vi "hickey_FinalProject.vi"() -> ()   [LabVIEW 2014]
uses:
  <vilib>/MakerHub/LINX/Private/Type Defs/User Platform.ctl
  <vilib>/MakerHub/LINX/Private/Type Defs/Interface.ctl
  <vilib>/MakerHub/LINX/Public/Peripherals/Analog/Analog Read 1 Chan.vi
  <vilib>/MakerHub/LINX/Public/Peripherals/Digital/Digital Write 1 Chan.vi
  <vilib>/MakerHub/LINX/LMH-LINX.lvlib
panel:
  out "AI Value":dbl
  in  "Serial Port":refnum<visa-resource-name>="N/A"
  in  "Interface":T1
  in  "Platform":T2
  in  "stop":bool
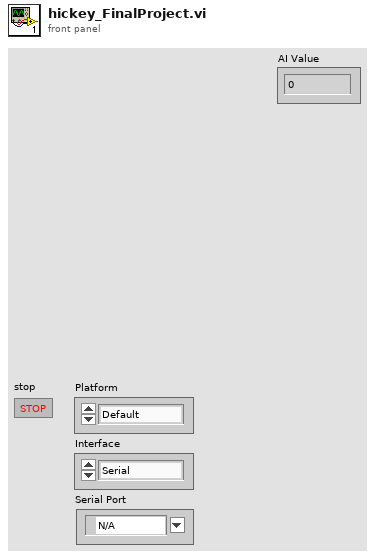
[diagram p1: front panel]
types:
  T1 = typedef "LMH-LINX.lvlib/Interface.ctl" = enum16{"Serial", "TCP"}
  T2 = typedef "LMH-LINX.lvlib/User Platform.ctl" = enum16{"Default", "LINX", "myRIO"}
  T3 = typedef "LMH-LINX.lvlib/LINX Ref.ctl" = cluster{"Platform":T4, "Interface":T1, "LINX Device Config":T5}
  T4 = typedef "LMH-LINX.lvlib/Platform.ctl" = enum16{"LINX", "myRIO"}
  T5 = typedef "LMH-LINX.lvlib/Device.lvlib/LINX Device Config.ctl" = cluster{"Interface":T1, "COM Port":refnum<visa-resource-name>, "TCP Configuration":T6, "Device Family":u8, "Device ID":u8, "Device Name":string, "TCP Ref":refnum<k5>, "Channels":T7}
  T6 = typedef "LMH-LINX.lvlib/Device.lvlib/TCP Config.ctl" = cluster{"IP Address":string, "Port":u16}
  T7 = typedef "LMH-LINX.lvlib/Channels.ctl" = cluster{"DI":u8[], "DO":u8[], "AI":u8[], "AO":u8[], "PWM":u8[], "QE":u8[], "UART":u8[], "I2C 2":u8[], "SPI":u8[], "CAN":u8[], "Servo":u8[], "AI Ref (V)":dbl, "AO Ref (V)":dbl, "AO Resolution (Bits)":u8}
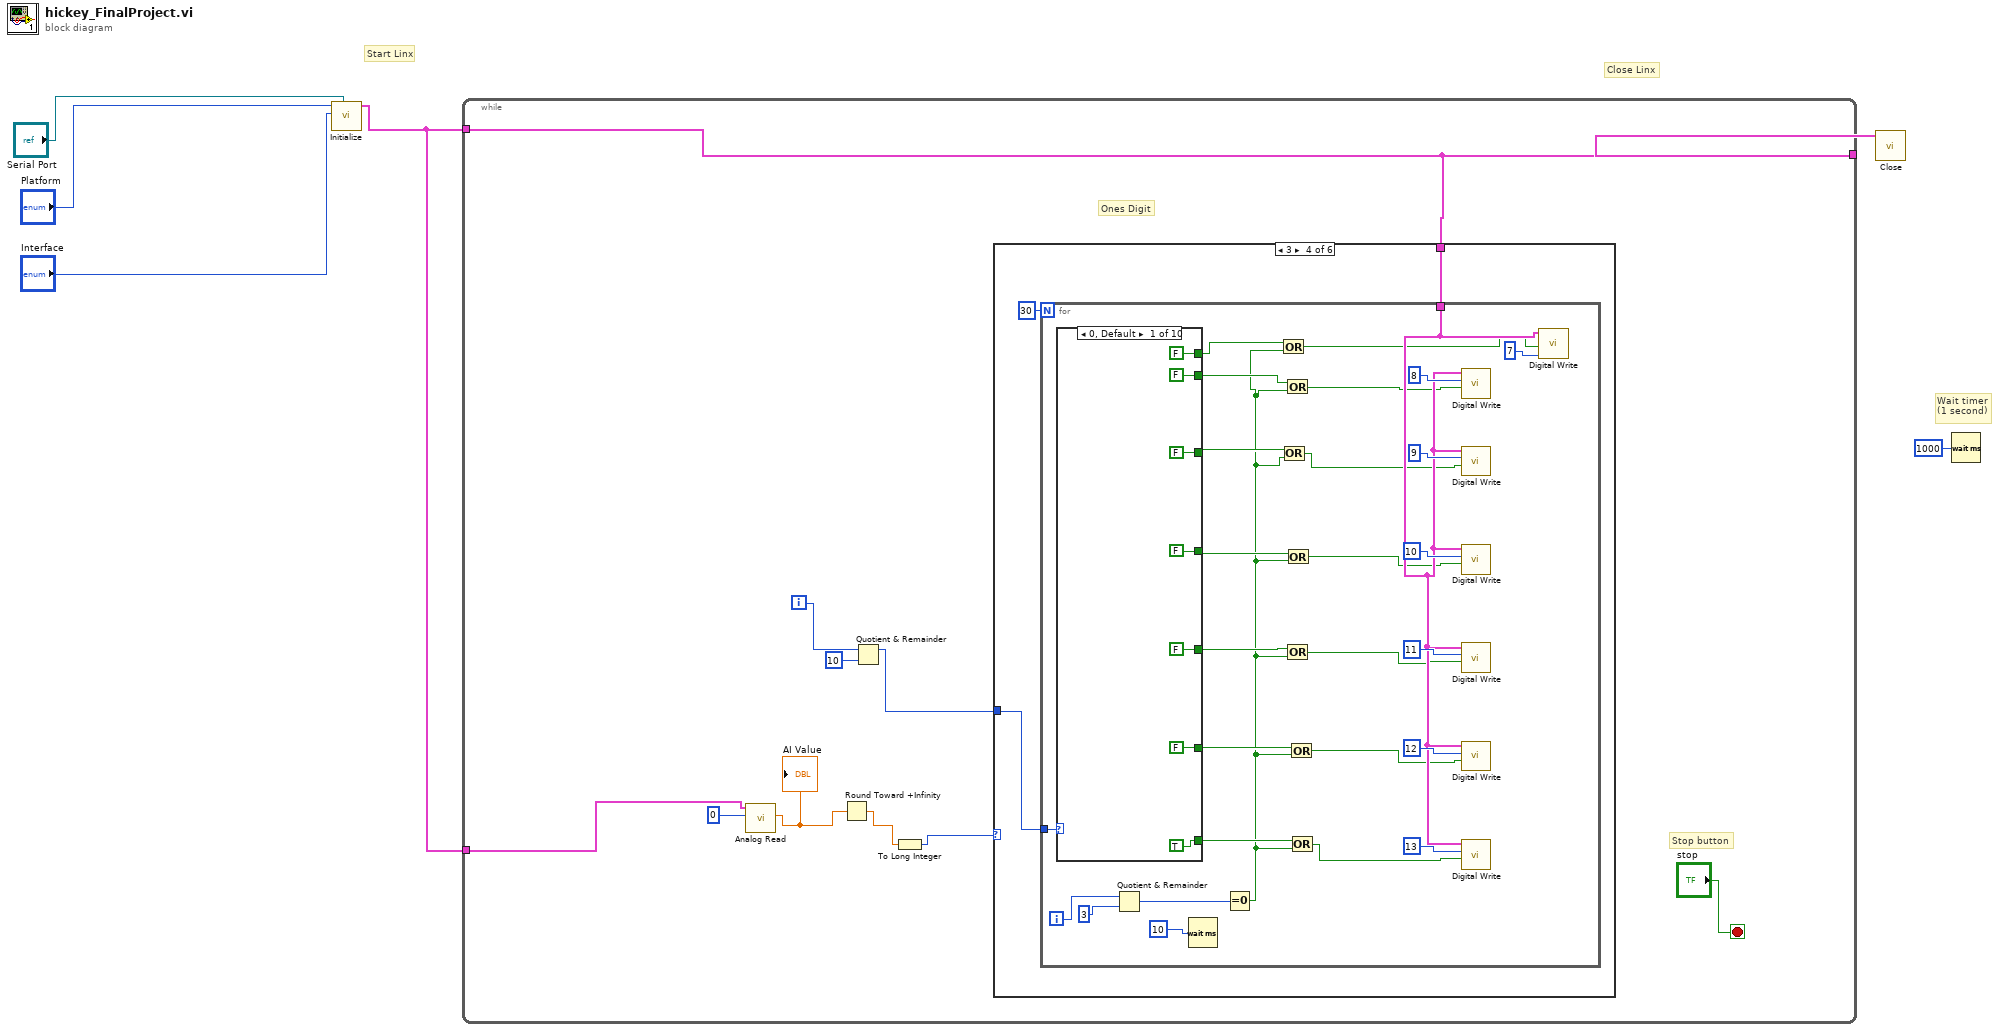
[diagram p0: block diagram]
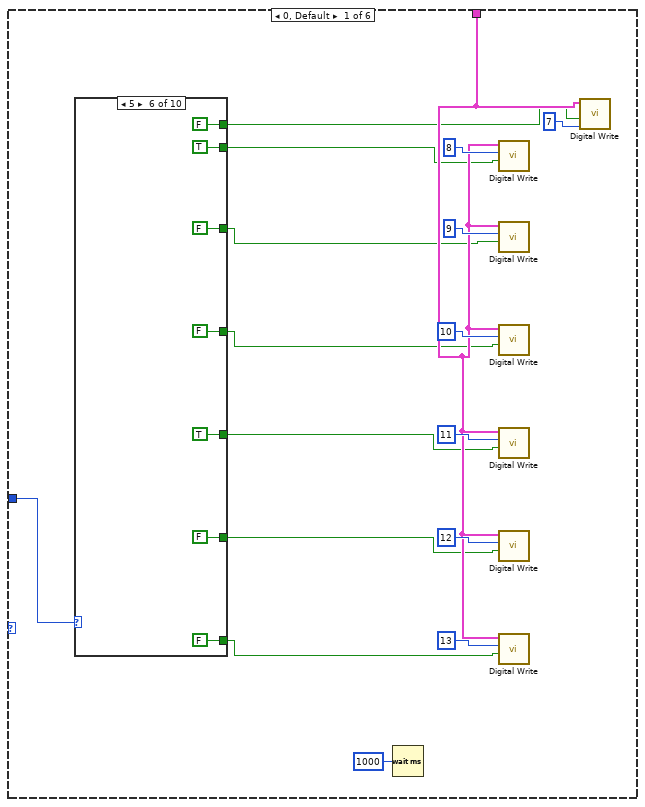
[diagram p2: hidden frame]
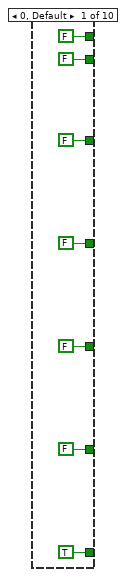
[diagram p3: hidden frame]
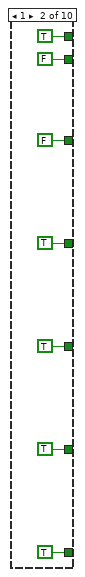
[diagram p4: hidden frame]
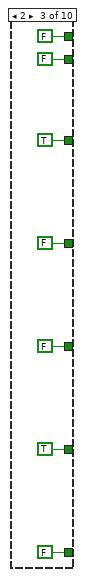
[diagram p5: hidden frame]
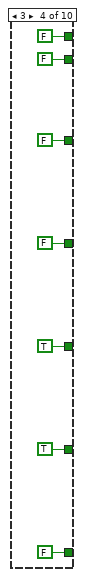
[diagram p6: hidden frame]
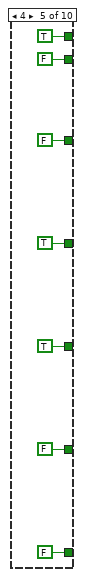
[diagram p7: hidden frame]
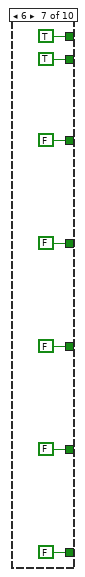
[diagram p8: hidden frame]
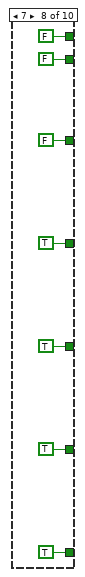
[diagram p9: hidden frame]
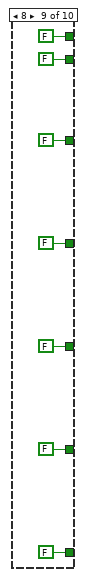
[diagram p10: hidden frame]
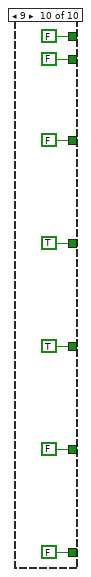
[diagram p11: hidden frame]
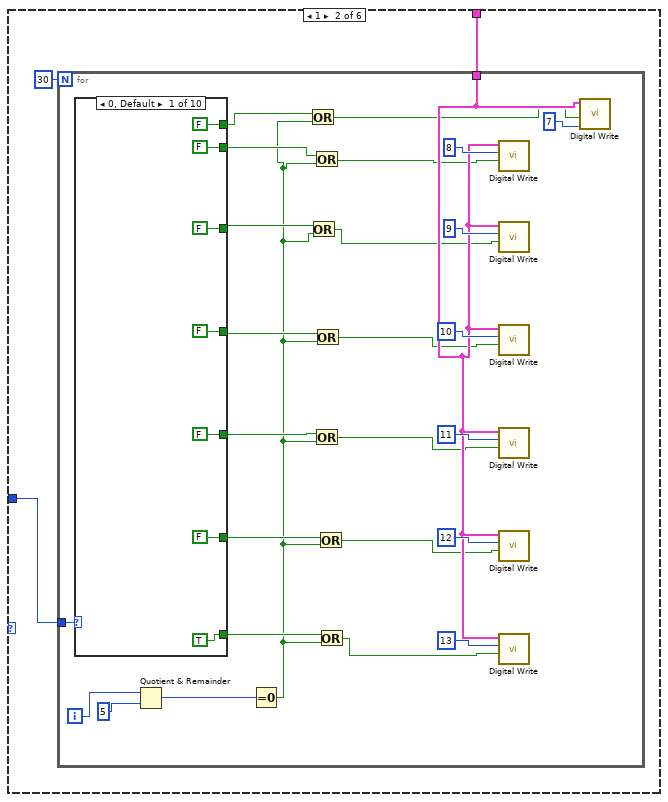
[diagram p12: hidden frame]
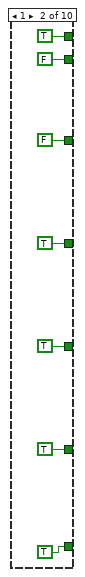
[diagram p13: hidden frame]
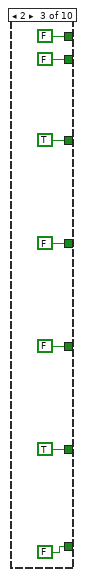
[diagram p14: hidden frame]
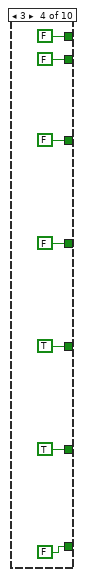
[diagram p15: hidden frame]
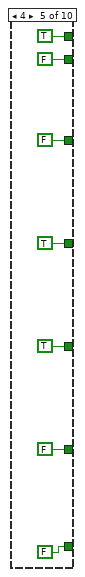
[diagram p16: hidden frame]
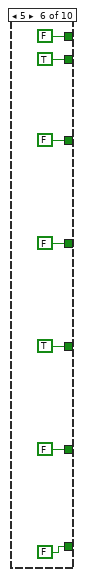
[diagram p17: hidden frame]
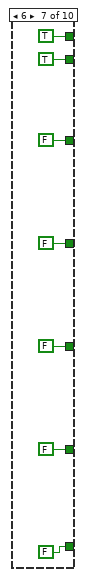
[diagram p18: hidden frame]
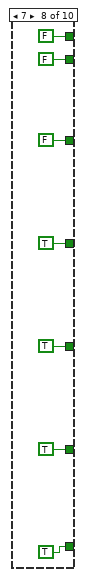
[diagram p19: hidden frame]
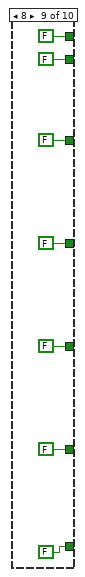
[diagram p20: hidden frame]
diagram:
  # "Wait timer\n(1 second)"
  # "Close Linx"
  # "Start Linx"
  n1 = call <vilib>:"Initialize.vi"("Serial Port"="Serial Port", "Interface"="Interface", "Platform"="Platform") -> ("LINX Ref"=w2:T3)  [unwired: 6 in, 2 out]
  n2 = while {
    tunnel: [w15] -> w6
    tunnel: w2 -> [w15]
    tunnel: w2 -> [w10]
    i -> [w14]
    stop <- "stop" stop-if-true
    # "Stop button"
    # "Ones Digit"
    n3 = call-poly <vilib>:"Analog Read.vi"("Analog Channel"=u8 0, "LINX Resource"=w10) -> ("AI Value"=w8:dbl)  [unwired: 6 in, 3 out]
    "AI Value" <- w8
    n4 = Round Toward +Infinity(x=w8) -> (ceil(x): smallest int >= x=w7:dbl)
    n5 = Quotient & Remainder(x=w14, y=10) -> (x-y*floor(x/y)=w12:i32)  [unwired: 1 out]
    n6 = To Long Integer(number=w7) -> (32bit integer=w9:i32)
    n7 = case shown="3" w9 {
      tunnel: w15 -> [w26 w106 w206 w307 w408 w516]
      tunnel: w12 -> [w17 w104 w204 w305 w407 w507]
      frame 0, Default {
        n8 = case shown="5" w17 {
          tunnel: [FALSE FALSE FALSE FALSE FALSE TRUE TRUE FALSE FALSE FALSE] -> w24
          tunnel: [FALSE FALSE TRUE FALSE FALSE FALSE FALSE FALSE FALSE FALSE] -> w23
          tunnel: [FALSE TRUE FALSE FALSE TRUE FALSE FALSE TRUE FALSE TRUE] -> w22
          tunnel: [FALSE TRUE FALSE TRUE TRUE TRUE FALSE TRUE FALSE TRUE] -> w21
          tunnel: [FALSE TRUE TRUE TRUE FALSE FALSE FALSE TRUE FALSE FALSE] -> w20
          tunnel: [FALSE TRUE FALSE FALSE TRUE FALSE TRUE FALSE FALSE FALSE] -> w25
          tunnel: [TRUE TRUE FALSE FALSE FALSE FALSE FALSE TRUE FALSE FALSE] -> w19
          frame 0, Default {
          }
          frame 1 {
          }
          frame 2 {
          }
          frame 3 {
          }
          frame 4 {
          }
          frame 5 {
          }
          frame 6 {
          }
          frame 7 {
          }
          frame 8 {
          }
          frame 9 {
          }
        }
        n9 = Wait (ms)(milliseconds to wait=u32 1000) -> ()  [unwired: 1 out]
        n10 = call-poly <vilib>:"Digital Write.vi"("Output Value"=w24, "DO Channel"=u8 8, "LINX Resource"=w26) -> ()  [unwired: 7 in, 2 out]
        n11 = call-poly <vilib>:"Digital Write.vi"("Output Value"=w23, "DO Channel"=u8 9, "LINX Resource"=w26) -> ()  [unwired: 7 in, 2 out]
        n12 = call-poly <vilib>:"Digital Write.vi"("Output Value"=w22, "DO Channel"=u8 10, "LINX Resource"=w26) -> ()  [unwired: 7 in, 2 out]
        n13 = call-poly <vilib>:"Digital Write.vi"("Output Value"=w21, "DO Channel"=u8 11, "LINX Resource"=w26) -> ()  [unwired: 7 in, 2 out]
        n14 = call-poly <vilib>:"Digital Write.vi"("Output Value"=w20, "DO Channel"=u8 12, "LINX Resource"=w26) -> ()  [unwired: 7 in, 2 out]
        n15 = call-poly <vilib>:"Digital Write.vi"("Output Value"=w19, "DO Channel"=u8 13, "LINX Resource"=w26) -> ()  [unwired: 7 in, 2 out]
        n16 = call-poly <vilib>:"Digital Write.vi"("Output Value"=w25, "DO Channel"=u8 7, "LINX Resource"=w26) -> ()  [unwired: 7 in, 2 out]
      }
      frame 1 {
        n17 = for {
          N: 30 -> [_]
          tunnel: w106 -> [w126]
          tunnel: w104 -> [w107]
          i -> [w125]
          n18 = case shown="0, Default" w107 {
            tunnel: [FALSE FALSE FALSE FALSE FALSE TRUE TRUE FALSE FALSE FALSE] -> w117
            tunnel: [FALSE FALSE TRUE FALSE FALSE FALSE FALSE FALSE FALSE FALSE] -> w118
            tunnel: [FALSE TRUE FALSE FALSE TRUE FALSE FALSE TRUE FALSE TRUE] -> w119
            tunnel: [FALSE TRUE FALSE TRUE TRUE TRUE FALSE TRUE FALSE TRUE] -> w120
            tunnel: [FALSE TRUE TRUE TRUE FALSE FALSE FALSE TRUE FALSE FALSE] -> w121
            tunnel: [FALSE TRUE FALSE FALSE TRUE FALSE TRUE FALSE FALSE FALSE] -> w116
            tunnel: [TRUE TRUE FALSE FALSE FALSE FALSE FALSE TRUE FALSE FALSE] -> w122
            frame 0, Default {
            }
            frame 1 {
            }
            frame 2 {
            }
            frame 3 {
            }
            frame 4 {
            }
            frame 5 {
            }
            frame 6 {
            }
            frame 7 {
            }
            frame 8 {
            }
            frame 9 {
            }
          }
          n19 = Quotient & Remainder(x=w125, y=5) -> (x-y*floor(x/y)=w123:i32)  [unwired: 1 out]
          n20 = Equal To 0?(x=w123) -> (x = 0?=w108:bool)
          n21 = Or(x=w116, y=w108) -> (x .or. y?=w109:bool)
          n22 = Or(x=w118, y=w108) -> (x .or. y?=w111:bool)
          n23 = Or(x=w117, y=w108) -> (x .or. y?=w110:bool)
          n24 = Or(x=w120, y=w108) -> (x .or. y?=w113:bool)
          n25 = Or(x=w119, y=w108) -> (x .or. y?=w112:bool)
          n26 = Or(x=w121, y=w108) -> (x .or. y?=w114:bool)
          n27 = Or(x=w122, y=w108) -> (x .or. y?=w115:bool)
          n28 = call-poly <vilib>:"Digital Write.vi"("Output Value"=w110, "DO Channel"=u8 8, "LINX Resource"=w126) -> ()  [unwired: 7 in, 2 out]
          n29 = call-poly <vilib>:"Digital Write.vi"("Output Value"=w111, "DO Channel"=u8 9, "LINX Resource"=w126) -> ()  [unwired: 7 in, 2 out]
          n30 = call-poly <vilib>:"Digital Write.vi"("Output Value"=w112, "DO Channel"=u8 10, "LINX Resource"=w126) -> ()  [unwired: 7 in, 2 out]
          n31 = call-poly <vilib>:"Digital Write.vi"("Output Value"=w113, "DO Channel"=u8 11, "LINX Resource"=w126) -> ()  [unwired: 7 in, 2 out]
          n32 = call-poly <vilib>:"Digital Write.vi"("Output Value"=w114, "DO Channel"=u8 12, "LINX Resource"=w126) -> ()  [unwired: 7 in, 2 out]
          n33 = call-poly <vilib>:"Digital Write.vi"("Output Value"=w115, "DO Channel"=u8 13, "LINX Resource"=w126) -> ()  [unwired: 7 in, 2 out]
          n34 = call-poly <vilib>:"Digital Write.vi"("Output Value"=w109, "DO Channel"=u8 7, "LINX Resource"=w126) -> ()  [unwired: 7 in, 2 out]
        }
      }
      frame 2 {
        n35 = for {
          N: 30 -> [_]
          tunnel: w206 -> [w227]
          tunnel: w204 -> [w208]
          i -> [w226]
          n36 = case shown="0, Default" w208 {
            tunnel: [FALSE FALSE FALSE FALSE FALSE TRUE TRUE FALSE FALSE FALSE] -> w218
            tunnel: [FALSE FALSE TRUE FALSE FALSE FALSE FALSE FALSE FALSE FALSE] -> w219
            tunnel: [FALSE TRUE FALSE FALSE TRUE FALSE FALSE TRUE FALSE TRUE] -> w220
            tunnel: [FALSE TRUE FALSE TRUE TRUE TRUE FALSE TRUE FALSE TRUE] -> w221
            tunnel: [FALSE TRUE TRUE TRUE FALSE FALSE FALSE TRUE FALSE FALSE] -> w222
            tunnel: [FALSE TRUE FALSE FALSE TRUE FALSE TRUE FALSE FALSE FALSE] -> w217
            tunnel: [TRUE TRUE FALSE FALSE FALSE FALSE FALSE TRUE FALSE FALSE] -> w223
            frame 0, Default {
            }
            frame 1 {
            }
            frame 2 {
            }
            frame 3 {
            }
            frame 4 {
            }
            frame 5 {
            }
            frame 6 {
            }
            frame 7 {
            }
            frame 8 {
            }
            frame 9 {
            }
          }
          n37 = Quotient & Remainder(x=w226, y=4) -> (x-y*floor(x/y)=w224:i32)  [unwired: 1 out]
          n38 = Equal To 0?(x=w224) -> (x = 0?=w209:bool)
          n39 = Or(x=w217, y=w209) -> (x .or. y?=w210:bool)
          n40 = Or(x=w219, y=w209) -> (x .or. y?=w212:bool)
          n41 = Or(x=w218, y=w209) -> (x .or. y?=w211:bool)
          n42 = Or(x=w221, y=w209) -> (x .or. y?=w214:bool)
          n43 = Or(x=w220, y=w209) -> (x .or. y?=w213:bool)
          n44 = Or(x=w222, y=w209) -> (x .or. y?=w215:bool)
          n45 = Or(x=w223, y=w209) -> (x .or. y?=w216:bool)
          n46 = Wait (ms)(milliseconds to wait=u32 10) -> ()  [unwired: 1 out]
          n47 = call-poly <vilib>:"Digital Write.vi"("Output Value"=w211, "DO Channel"=u8 8, "LINX Resource"=w227) -> ()  [unwired: 7 in, 2 out]
          n48 = call-poly <vilib>:"Digital Write.vi"("Output Value"=w212, "DO Channel"=u8 9, "LINX Resource"=w227) -> ()  [unwired: 7 in, 2 out]
          n49 = call-poly <vilib>:"Digital Write.vi"("Output Value"=w213, "DO Channel"=u8 10, "LINX Resource"=w227) -> ()  [unwired: 7 in, 2 out]
          n50 = call-poly <vilib>:"Digital Write.vi"("Output Value"=w214, "DO Channel"=u8 11, "LINX Resource"=w227) -> ()  [unwired: 7 in, 2 out]
          n51 = call-poly <vilib>:"Digital Write.vi"("Output Value"=w215, "DO Channel"=u8 12, "LINX Resource"=w227) -> ()  [unwired: 7 in, 2 out]
          n52 = call-poly <vilib>:"Digital Write.vi"("Output Value"=w216, "DO Channel"=u8 13, "LINX Resource"=w227) -> ()  [unwired: 7 in, 2 out]
          n53 = call-poly <vilib>:"Digital Write.vi"("Output Value"=w210, "DO Channel"=u8 7, "LINX Resource"=w227) -> ()  [unwired: 7 in, 2 out]
        }
      }
      frame 3 {
        n54 = for {
          N: 30 -> [_]
          tunnel: w307 -> [w328]
          tunnel: w305 -> [w309]
          i -> [w327]
          n55 = case shown="0, Default" w309 {
            tunnel: [FALSE FALSE FALSE FALSE FALSE TRUE TRUE FALSE FALSE FALSE] -> w319
            tunnel: [FALSE FALSE TRUE FALSE FALSE FALSE FALSE FALSE FALSE FALSE] -> w320
            tunnel: [FALSE TRUE FALSE FALSE TRUE FALSE FALSE TRUE FALSE TRUE] -> w321
            tunnel: [FALSE TRUE FALSE TRUE TRUE TRUE FALSE TRUE FALSE TRUE] -> w322
            tunnel: [FALSE TRUE TRUE TRUE FALSE FALSE FALSE TRUE FALSE FALSE] -> w323
            tunnel: [FALSE TRUE FALSE FALSE TRUE FALSE TRUE FALSE FALSE FALSE] -> w318
            tunnel: [TRUE TRUE FALSE FALSE FALSE FALSE FALSE TRUE FALSE FALSE] -> w324
            frame 0, Default {
            }
            frame 1 {
            }
            frame 2 {
            }
            frame 3 {
            }
            frame 4 {
            }
            frame 5 {
            }
            frame 6 {
            }
            frame 7 {
            }
            frame 8 {
            }
            frame 9 {
            }
          }
          n56 = Quotient & Remainder(x=w327, y=3) -> (x-y*floor(x/y)=w325:i32)  [unwired: 1 out]
          n57 = Wait (ms)(milliseconds to wait=u32 10) -> ()  [unwired: 1 out]
          n58 = Equal To 0?(x=w325) -> (x = 0?=w310:bool)
          n59 = Or(x=w318, y=w310) -> (x .or. y?=w311:bool)
          n60 = Or(x=w320, y=w310) -> (x .or. y?=w313:bool)
          n61 = Or(x=w319, y=w310) -> (x .or. y?=w312:bool)
          n62 = Or(x=w322, y=w310) -> (x .or. y?=w315:bool)
          n63 = Or(x=w321, y=w310) -> (x .or. y?=w314:bool)
          n64 = Or(x=w323, y=w310) -> (x .or. y?=w316:bool)
          n65 = Or(x=w324, y=w310) -> (x .or. y?=w317:bool)
          n66 = call-poly <vilib>:"Digital Write.vi"("Output Value"=w312, "DO Channel"=u8 8, "LINX Resource"=w328) -> ()  [unwired: 7 in, 2 out]
          n67 = call-poly <vilib>:"Digital Write.vi"("Output Value"=w313, "DO Channel"=u8 9, "LINX Resource"=w328) -> ()  [unwired: 7 in, 2 out]
          n68 = call-poly <vilib>:"Digital Write.vi"("Output Value"=w314, "DO Channel"=u8 10, "LINX Resource"=w328) -> ()  [unwired: 7 in, 2 out]
          n69 = call-poly <vilib>:"Digital Write.vi"("Output Value"=w315, "DO Channel"=u8 11, "LINX Resource"=w328) -> ()  [unwired: 7 in, 2 out]
          n70 = call-poly <vilib>:"Digital Write.vi"("Output Value"=w316, "DO Channel"=u8 12, "LINX Resource"=w328) -> ()  [unwired: 7 in, 2 out]
          n71 = call-poly <vilib>:"Digital Write.vi"("Output Value"=w317, "DO Channel"=u8 13, "LINX Resource"=w328) -> ()  [unwired: 7 in, 2 out]
          n72 = call-poly <vilib>:"Digital Write.vi"("Output Value"=w311, "DO Channel"=u8 7, "LINX Resource"=w328) -> ()  [unwired: 7 in, 2 out]
        }
      }
      frame 4 {
        n73 = for {
          N: 30 -> [_]
          tunnel: w408 -> [w429]
          tunnel: w407 -> [w412]
          i -> [w428]
          n74 = case shown="0, Default" w412 {
            tunnel: [FALSE FALSE FALSE FALSE FALSE TRUE TRUE FALSE FALSE FALSE] -> w422
            tunnel: [FALSE FALSE TRUE FALSE FALSE FALSE FALSE FALSE FALSE FALSE] -> w423
            tunnel: [FALSE TRUE FALSE FALSE TRUE FALSE FALSE TRUE FALSE TRUE] -> w424
            tunnel: [FALSE TRUE FALSE TRUE TRUE TRUE FALSE TRUE FALSE TRUE] -> w425
            tunnel: [FALSE TRUE TRUE TRUE FALSE FALSE FALSE TRUE FALSE FALSE] -> w426
            tunnel: [FALSE TRUE FALSE FALSE TRUE FALSE TRUE FALSE FALSE FALSE] -> w421
            tunnel: [TRUE TRUE FALSE FALSE FALSE FALSE FALSE TRUE FALSE FALSE] -> w427
            frame 0, Default {
            }
            frame 1 {
            }
            frame 2 {
            }
            frame 3 {
            }
            frame 4 {
            }
            frame 5 {
            }
            frame 6 {
            }
            frame 7 {
            }
            frame 8 {
            }
            frame 9 {
            }
          }
          n75 = Quotient & Remainder(x=w428, y=2) -> (x-y*floor(x/y)=w411:i32)  [unwired: 1 out]
          n76 = Wait (ms)(milliseconds to wait=u32 10) -> ()  [unwired: 1 out]
          n77 = Equal To 0?(x=w411) -> (x = 0?=w413:bool)
          n78 = Or(x=w421, y=w413) -> (x .or. y?=w414:bool)
          n79 = Or(x=w423, y=w413) -> (x .or. y?=w416:bool)
          n80 = Or(x=w422, y=w413) -> (x .or. y?=w415:bool)
          n81 = Or(x=w425, y=w413) -> (x .or. y?=w418:bool)
          n82 = Or(x=w424, y=w413) -> (x .or. y?=w417:bool)
          n83 = Or(x=w426, y=w413) -> (x .or. y?=w419:bool)
          n84 = Or(x=w427, y=w413) -> (x .or. y?=w420:bool)
          n85 = call-poly <vilib>:"Digital Write.vi"("Output Value"=w415, "DO Channel"=u8 8, "LINX Resource"=w429) -> ()  [unwired: 7 in, 2 out]
          n86 = call-poly <vilib>:"Digital Write.vi"("Output Value"=w416, "DO Channel"=u8 9, "LINX Resource"=w429) -> ()  [unwired: 7 in, 2 out]
          n87 = call-poly <vilib>:"Digital Write.vi"("Output Value"=w417, "DO Channel"=u8 10, "LINX Resource"=w429) -> ()  [unwired: 7 in, 2 out]
          n88 = call-poly <vilib>:"Digital Write.vi"("Output Value"=w418, "DO Channel"=u8 11, "LINX Resource"=w429) -> ()  [unwired: 7 in, 2 out]
          n89 = call-poly <vilib>:"Digital Write.vi"("Output Value"=w419, "DO Channel"=u8 12, "LINX Resource"=w429) -> ()  [unwired: 7 in, 2 out]
          n90 = call-poly <vilib>:"Digital Write.vi"("Output Value"=w420, "DO Channel"=u8 13, "LINX Resource"=w429) -> ()  [unwired: 7 in, 2 out]
          n91 = call-poly <vilib>:"Digital Write.vi"("Output Value"=w414, "DO Channel"=u8 7, "LINX Resource"=w429) -> ()  [unwired: 7 in, 2 out]
        }
      }
      frame 5 {
        n92 = case shown="0, Default" w507 {
          tunnel: [FALSE FALSE FALSE FALSE FALSE TRUE TRUE FALSE FALSE FALSE] -> w514
          tunnel: [FALSE FALSE TRUE FALSE FALSE FALSE FALSE FALSE FALSE FALSE] -> w513
          tunnel: [FALSE TRUE FALSE FALSE TRUE FALSE FALSE TRUE FALSE TRUE] -> w512
          tunnel: [FALSE TRUE FALSE TRUE TRUE TRUE FALSE TRUE FALSE TRUE] -> w511
          tunnel: [FALSE TRUE TRUE TRUE FALSE FALSE FALSE TRUE FALSE FALSE] -> w510
          tunnel: [FALSE TRUE FALSE FALSE TRUE FALSE TRUE FALSE FALSE FALSE] -> w515
          tunnel: [TRUE TRUE FALSE FALSE FALSE FALSE FALSE TRUE FALSE FALSE] -> w509
          frame 0, Default {
          }
          frame 1 {
          }
          frame 2 {
          }
          frame 3 {
          }
          frame 4 {
          }
          frame 5 {
          }
          frame 6 {
          }
          frame 7 {
          }
          frame 8 {
          }
          frame 9 {
          }
        }
        n93 = Wait (ms)(milliseconds to wait=u32 1000) -> ()  [unwired: 1 out]
        n94 = call-poly <vilib>:"Digital Write.vi"("Output Value"=w514, "DO Channel"=u8 8, "LINX Resource"=w516) -> ()  [unwired: 7 in, 2 out]
        n95 = call-poly <vilib>:"Digital Write.vi"("Output Value"=w513, "DO Channel"=u8 9, "LINX Resource"=w516) -> ()  [unwired: 7 in, 2 out]
        n96 = call-poly <vilib>:"Digital Write.vi"("Output Value"=w512, "DO Channel"=u8 10, "LINX Resource"=w516) -> ()  [unwired: 7 in, 2 out]
        n97 = call-poly <vilib>:"Digital Write.vi"("Output Value"=w511, "DO Channel"=u8 11, "LINX Resource"=w516) -> ()  [unwired: 7 in, 2 out]
        n98 = call-poly <vilib>:"Digital Write.vi"("Output Value"=w510, "DO Channel"=u8 12, "LINX Resource"=w516) -> ()  [unwired: 7 in, 2 out]
        n99 = call-poly <vilib>:"Digital Write.vi"("Output Value"=w509, "DO Channel"=u8 13, "LINX Resource"=w516) -> ()  [unwired: 7 in, 2 out]
        n100 = call-poly <vilib>:"Digital Write.vi"("Output Value"=w515, "DO Channel"=u8 7, "LINX Resource"=w516) -> ()  [unwired: 7 in, 2 out]
      }
    }
  }
  n101 = call <vilib>:"Close.vi"("LINX Resource"=w6) -> ()  [unwired: 9 in, 2 out]
  n102 = Wait (ms)(milliseconds to wait=u32 1000) -> ()  [unwired: 1 out]
